vi "Open Hardware.vi"(8 "error in (no error)":errorcluster, 11 "Instrument.SR7270 in":refnum<class "Instrument.SR7270.lvclass">) -> (0 "error out":errorcluster, 3 "Instrument.SR7270 out":refnum<class "Instrument.SR7270.lvclass">)   [LabVIEW 2019, in "Instrument.SR7270.lvclass"]
uses:
  Instrument.SR7270.lvclass
  C:/Program Files (x86)/National Instruments/LabVIEW 2019/user.lib/LevyLab/Instrument Framework/SMOs/Instrument/Instrument.lvclass
  <userlib>/LevyLab/Instrument Framework/SMOs/Instrument/Instrument.lvclass/Instrument.ctl
  Instrument.SR7270.lvclass/Instrument.SR7270.ctl
  Driver/SR7270 Drivers.lvlib
  <userlib>/LevyLab/Instrument Framework/SMOs/Instrument/Instrument.lvclass
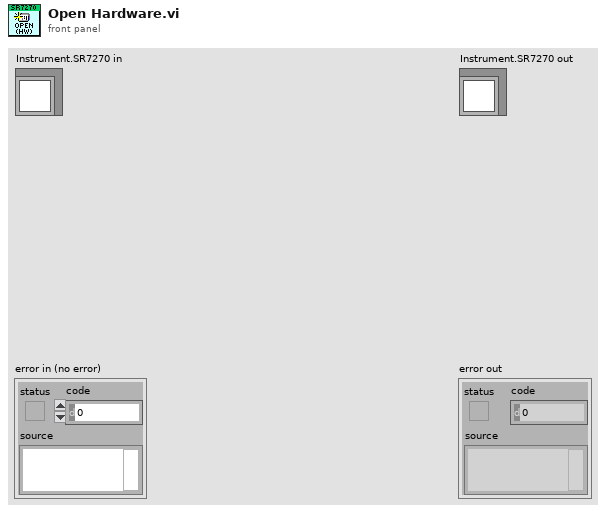
[diagram p1: front panel]
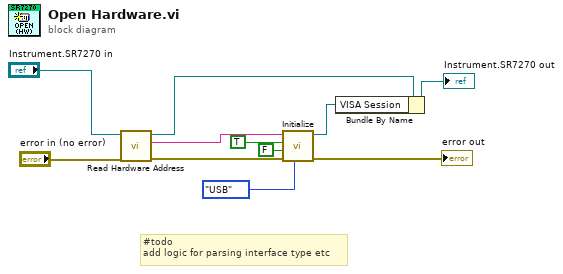
[diagram p0: block diagram]
diagram:
  # "#todo\nadd logic for parsing interface type etc"
  n1 = call <userlib>:"Read Hardware Address.vi"("error in (no error)"="error in (no error)", "Instrument in"="Instrument.SR7270 in") -> ("error out"=w8:errorcluster, "Address"=w5:string, "Instrument out"=w6:refnum<class "Instrument.SR7270.lvclass">)  [unwired: 7 in]
  n2 = call "Initialize.vi"("Interface"=enum16{"RS232", "USB", "Ethernet"}."USB", "error in (no error)"=w8, "reset"=FALSE, "ID query"=TRUE ("reset"), "Address"=w5) -> ("error out"=→"error out":errorcluster, "VISA resource name out"=w7:refnum<visa-resource-name>)  [unwired: 5 in]
  n3 = Bundle By Name(cluster=w6, "VISA Session"=w7) -> (→"Instrument.SR7270 out":refnum<class "Instrument.SR7270.lvclass">)
